vi "Perform Action.vi"(8 "error in (no error)":errorcluster, 10 "Input":variant, 11 "Virt Instrument Base in":refnum<class "Virt Voltage Generator.lvclass">) -> (0 "error out":errorcluster, 2 "Output":variant, 3 "Virt Instrument Base out":refnum<class "Virt Voltage Generator.lvclass">)   [LabVIEW 2023, in "Virt Instrs FGen.lvlib" / "Virt Voltage Generator.lvclass"]
uses:
  Virt Voltage Generator.lvclass
  Virt Voltage Generator.lvclass/Virt Voltage Generator.ctl
  Virt Instr Host/Virt Instr Local.lvclass
  Instrument/Instrument.lvclass
  FGen PXI/FGen PXI Std Waveform CFG/Std Waveform Action Pams.ctl
  FGen PXI/FGen PXI Std Waveform CFG/FGen PXI Std Waveform CFG.lvclass
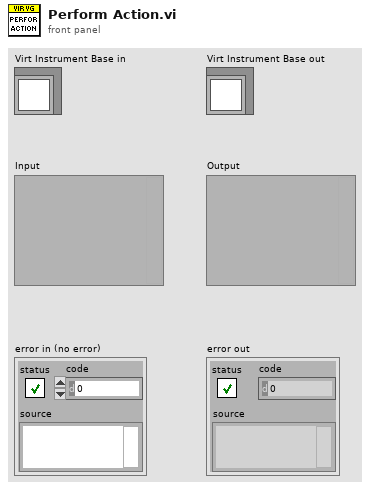
[diagram p1: front panel]
types:
  T1 = typedef "FGen PXI Std Waveform CFG.lvlib/FGen PXI Std Waveform CFG.lvclass/Std Waveform Action Pams.ctl" = cluster{"Frequency":dbl, "Amplitude":dbl, "DC Offset":dbl}
  T2 = cluster{"Channel":string, "Std Waveform Pams":T1}
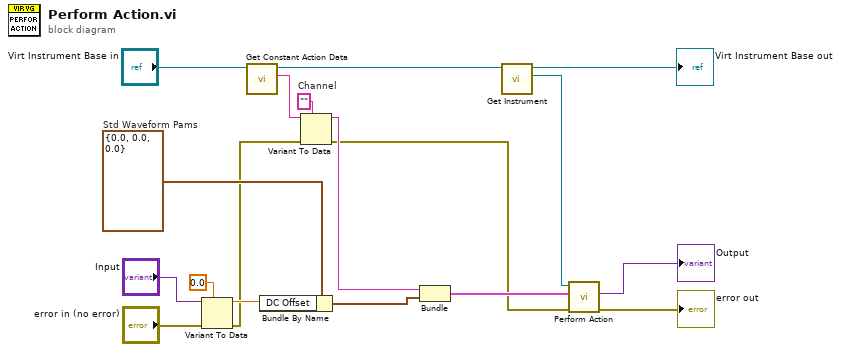
[diagram p0: block diagram]
diagram:
  w14 = ""  # Channel
  w5 = T1 {"Frequency"=0.0, "Amplitude"=0.0, "DC Offset"=0.0}  # Std Waveform Pams
  n1 = Variant To Data(error in="error in (no error)", type=0.0, Variant="Input") -> (data=w4:dbl, error out=w1:errorcluster)
  n2 = call "Get Constant Action Data.vi"("Virt Instr Base in"="Virt Instrument Base in") -> ("<JSON> Constant Action Data"=w13:string, "Virt Instr Base out"=w12:refnum<class "Virt Voltage Generator.lvclass">)  [unwired: 9 in]
  n3 = Bundle By Name(cluster=w5, "DC Offset"=w4) -> (w3:T1)
  n4 = Variant To Data(error in=w1, type=w14, Variant=w13) -> (data=w7:string, error out=w2:errorcluster)
  n5 = Bundle("Channel"=w7, "Std Waveform Pams"=w3) -> (w6:T2)  [unwired: 1 in]
  n6 = call "Get Instrument.vi"("Virt Instr Base in"=w12) -> ("HAL GOOP4.lvlib:Instrument"=w11:refnum<class "Instrument.lvclass">, "Virt Instr Base out"=→"Virt Instrument Base out":refnum<class "Virt Voltage Generator.lvclass">)  [unwired: 9 in]
  n7 = call "Perform Action.vi"("Error In"=w2, "Input"=w6, "reference in"=w11) -> ("Error Out"=→"error out":errorcluster, "Output"=→"Output":variant)  [unwired: 6 in, 1 out]
